vi "Validate Library.vi"(10 "Filename":string, 11 "path in":path) -> (1 "Full Path":path, 2 "valid":bool, 3 "Discovered Plugin":T1)   [LabVIEW 2021, in "CIFLauncher.lvclass"]
uses:
  CIFLauncher.lvclass
  CIFLauncher.lvclass/CIFLauncher.ctl
  <vilib>/Utility/LVLibp/NI_PackedLibraryUtility.lvlib
  CIFCore/Common/Typedef/Version.ctl
  CIFCore/Common/CIFCoreCommon.lvlib
  typedef/trash_Discovered Plugin.ctl
  typedef/trash_Plugin Metadata.ctl
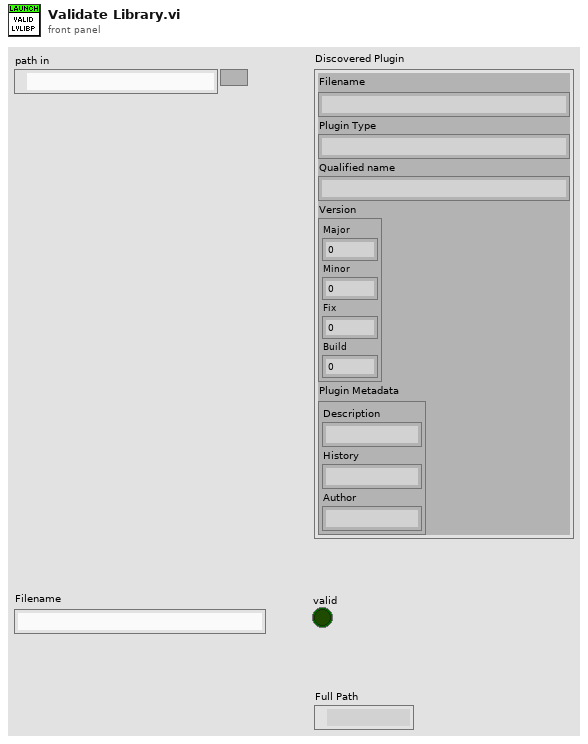
[diagram p1: front panel]
types:
  T1 = typedef "trash_Discovered Plugin.ctl" = cluster{"Filename":string, "Plugin Type":string, "Qualified name":string, "Version":T2, "Plugin Metadata":T3}
  T2 = typedef "CIFCoreCommon.lvlib/Version.ctl" = cluster{"Major":i32, "Minor":i32, "Fix":i32, "Build":i32}
  T3 = typedef "trash_Plugin Metadata.ctl" = cluster{"Description":string, "History":string, "Author":string}
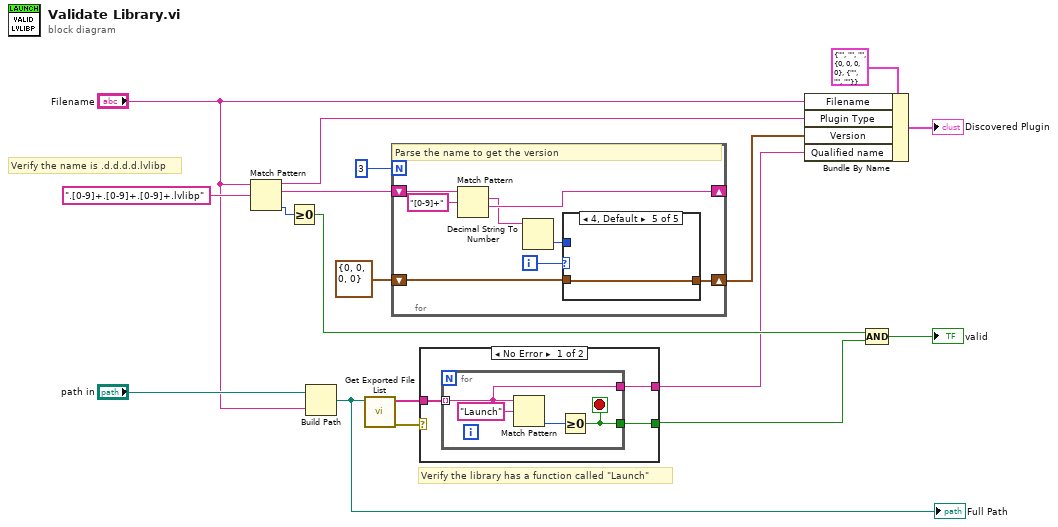
[diagram p0: block diagram]
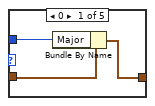
[diagram p2: hidden frame]
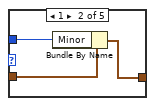
[diagram p3: hidden frame]
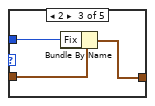
[diagram p4: hidden frame]
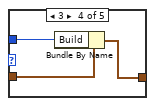
[diagram p5: hidden frame]
diagram:
  # "Verify the name is .d.d.d.d.lvlibp"
  # "Verify the library has a function called \"Launch\""
  n1 = Match Pattern(string="Filename", regular expression=".[0-9]+.[0-9]+.[0-9]+.lvlibp" ("Expression")) -> (before substring=w3:string, match substring=w14:string, offset past match=w9:i32)  [unwired: 1 in, 1 out]
  n2 = Greater Or Equal To 0?(x=w9) -> (x >= 0?=w7:bool)
  n3 = Build Path(base path="path in", name or relative path="Filename") -> (appended path=w1:path)
  "Full Path" <- w1
  n4 = call <vilib>:"Get Exported File List.vi"("packed library path"=w1) -> ("error out"=w18:errorcluster, "qualified names"=w17:string[])  [unwired: 8 in, 1 out]
  n5 = for {
    N: 3 -> [_]
    shift-right: [w24] -> _
    shift-left: w14 -> [w26]
    shift-right: [w19] -> w10
    shift-left: T2 {"Major"=0, "Minor"=0, "Fix"=0, "Build"=0} ("Version") -> [w22]
    i -> [w23]
    # "Parse the name to get the version"
    n6 = Match Pattern(string=w26, regular expression="[0-9]+") -> (match substring=w21:string, after substring=w24:string)  [unwired: 1 in, 2 out]
    n7 = Decimal String To Number(string=w21) -> (number=w20:i32)  [unwired: 2 in, 1 out]
    n8 = case shown="4, Default" w23 {
      tunnel: w22 -> [w29 w30 w33 w36 w39]
      tunnel: w20 -> [w28 w32 w35 w38 _]
      tunnel: [w27 w31 w34 w37 w39] -> w19
      frame 0 {
        n9 = Bundle By Name(cluster=w29, "Major"=w28) -> (w27:T2)
      }
      frame 1 {
        n10 = Bundle By Name(cluster=w30, "Minor"=w32) -> (w31:T2)
      }
      frame 2 {
        n11 = Bundle By Name(cluster=w33, "Fix"=w35) -> (w34:T2)
      }
      frame 3 {
        n12 = Bundle By Name(cluster=w36, "Build"=w38) -> (w37:T2)
      }
      frame 4, Default {
      }
    }
  }
  n13 = case shown="No Error" w18 {
    tunnel: w17 -> [w42 _]
    tunnel: [w41 _] -> w6
    tunnel: [w40 _] -> w2
    frame No Error {
      n14 = for {
        tunnel: w42 -> [w43] mode=indexing
        tunnel: [w44] -> w41
        tunnel: [w43] -> w40
        stop <- w44 stop-if-true
        n15 = Match Pattern(string=w43, regular expression="Launch") -> (offset past match=w45:i32)  [unwired: 1 in, 3 out]
        n16 = Greater Or Equal To 0?(x=w45) -> (x >= 0?=w44:bool)
      }
    }
    frame Error {
    }
  }
  n17 = Bundle By Name(cluster=T1 {"Filename"="", "Plugin Type"="", "Qualified name"="", "Version"={"Major"=0, "Minor"=0, "Fix"=0, "Build"=0}, "Plugin Metadata"={"Description"="", "History"="", "Author"=""}} ("Discovered Plugin"), "Filename"="Filename", "Plugin Type"=w3, "Version"=w10, "Qualified name"=w2) -> (→"Discovered Plugin":T1)
  n18 = Compound Arithmetic op=AND(w7, w6) -> (→"valid":bool)
